vi "Timing FGV.vi"() -> ()   [LabVIEW 2017]
panel:
  out "vergangene Zeit":dbl
  in  "Pause":bool=TRUE
  out "Time passed - Reset":bool
  in  "Zielzeit":dbl
  in  "Reset":bool=TRUE
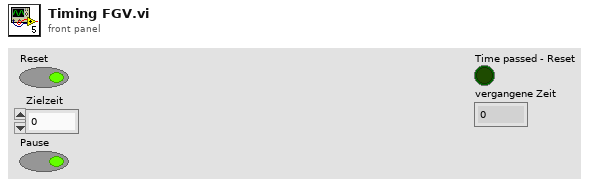
[diagram p1: front panel]
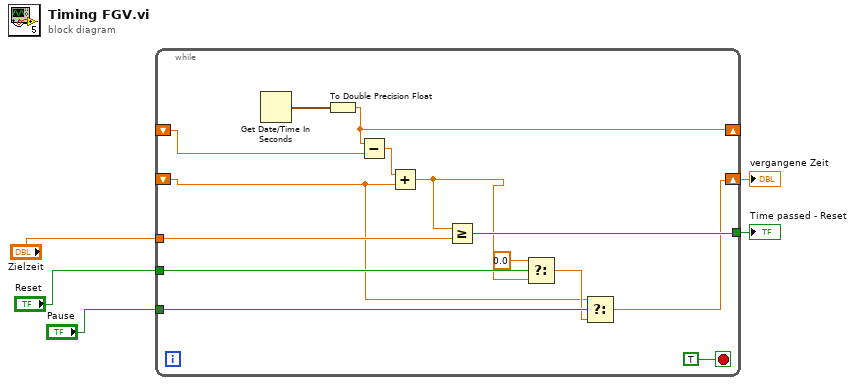
[diagram p0: block diagram]
diagram:
  n1 = while {
    shift-right: [w18] -> _
    shift-left: _ -> [w17]
    shift-right: [w7] -> w1
    shift-left: _ -> [w8]
    tunnel: "Zielzeit" -> [w15]
    tunnel: [w14] -> w4
    tunnel: "Reset" -> [w13]
    tunnel: "Pause" -> [w10]
    stop <- TRUE stop-if-true
    n2 = Get Date/Time In Seconds() -> (seconds since 1Jan1904=w19:timestamp)
    n3 = To Double Precision Float(number=w19) -> (double precision float=w18:dbl)
    n4 = Subtract(x=w18, y=w17) -> (x-y=w16:dbl)
    n5 = Add(x=w16, y=w8) -> (x+y=w11:dbl)
    n6 = Greater Or Equal?(x=w11, y=w15) -> (x >= y?=w14:bool)
    n7 = Select(t=0.0, s=w13, f=w11) -> (s? t:f=w9:dbl)
    n8 = Select(t=w8, s=w10, f=w9) -> (s? t:f=w7:dbl)
  }
  "Time passed - Reset" <- w4
  "vergangene Zeit" <- w1
